vi "Auto Build Script.vi"(8 "error in (no error)":errorcluster, 11 "PostBuildSupport":refnum<class "PostBuildSupport.lvclass">) -> (0 "error out":errorcluster)   [LabVIEW 2019, in "PostBuildSupport.lvclass"]
uses:
  PostBuildSupport.lvclass
  <userlib>/LevyLab/Progress Bar/ProgressBar/ProgressBar.lvclass
panel:
  in  "OK":bool
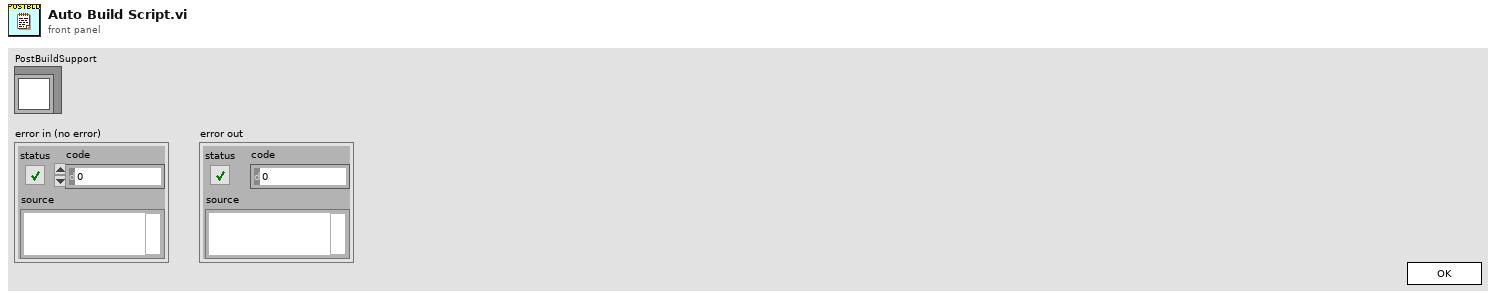
[diagram p1: front panel]
types:
  T1 = enum32{"Invalid", "Standard", "Closed", "Hidden", "Minimized", "Maximized"}
  T2 = enum32{"invalid app kind", "Development System", "Run Time System", "Student Edition", "Embedded LabVIEW", "Evaluation", "Custom"}
  T3 = cluster{"Core":cluster{"Current VI Reference":refnum<vi>, "Close Panel on Exit?":bool}, "PostBuildSupport":refnum<class "PostBuildSupport.lvclass">, "ProgressBar out":refnum<class "ProgressBar.lvclass">, "Progress Message":string, "Progress Bar":i32}
  T4 = cluster{"Current VI Reference":refnum<vi>, "Close Panel on Exit?":bool}
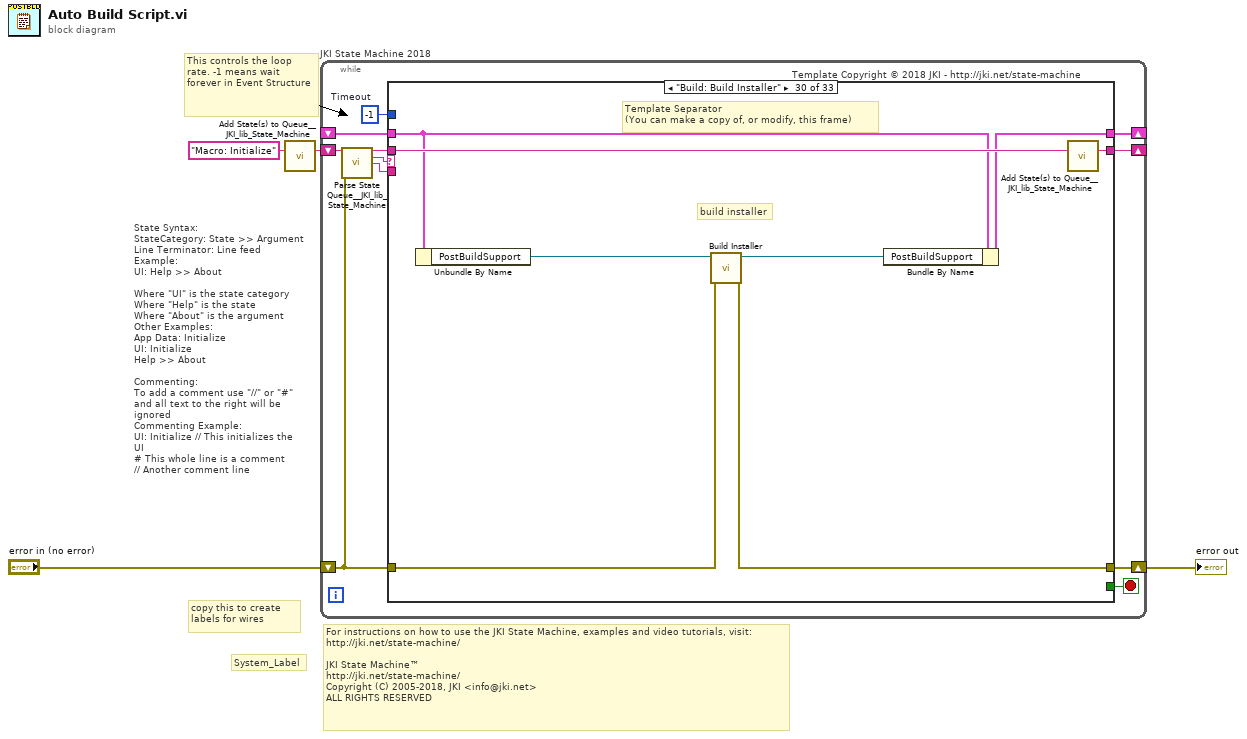
[diagram p0: block diagram]
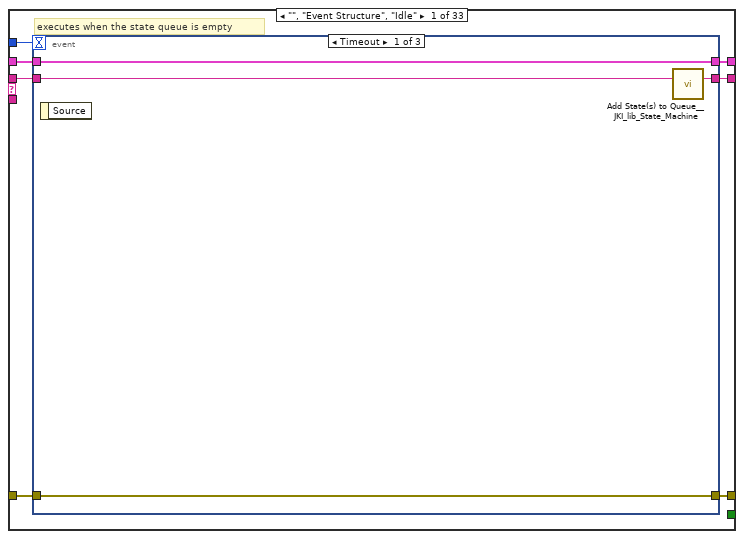
[diagram p2: hidden frame]
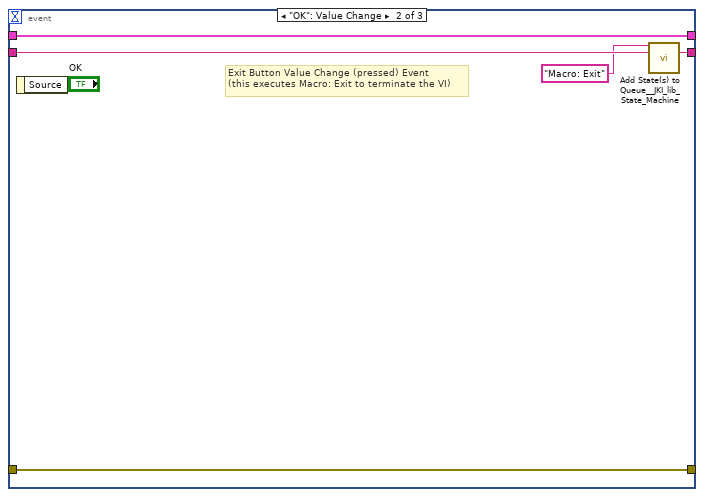
[diagram p3: hidden frame]
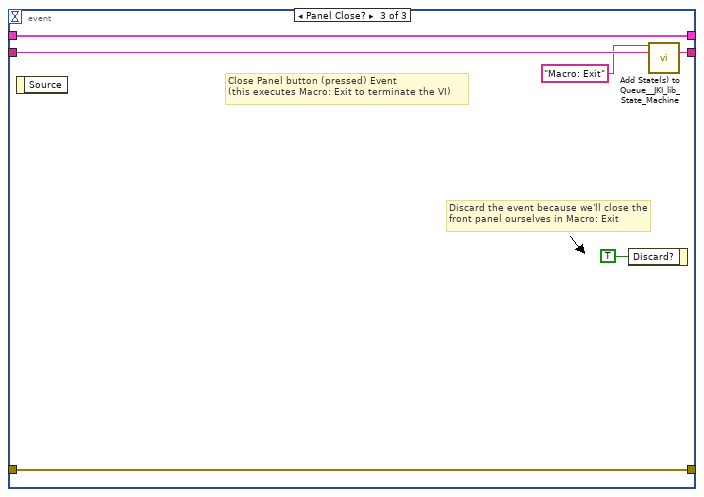
[diagram p4: hidden frame]
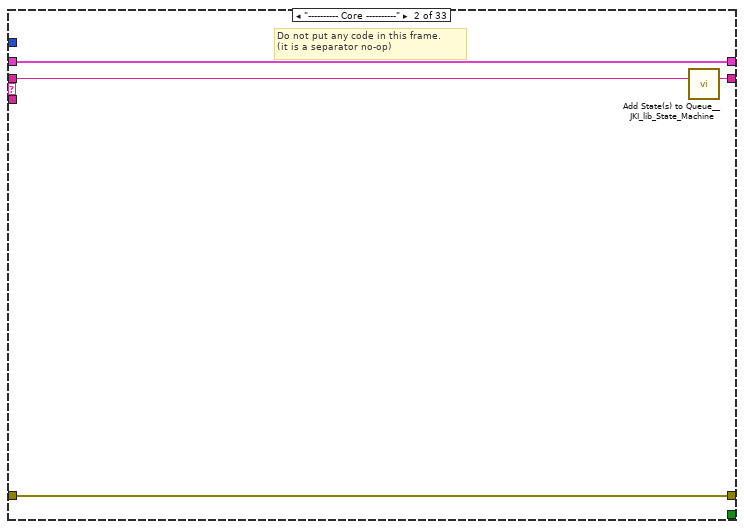
[diagram p5: hidden frame]
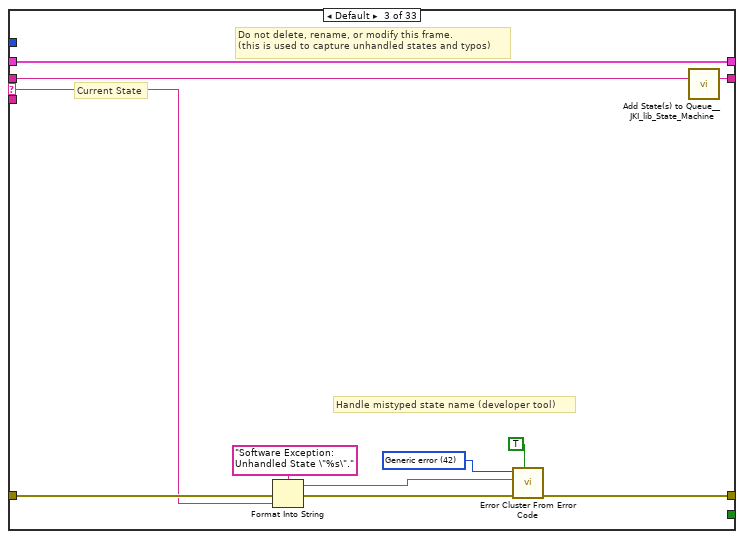
[diagram p6: hidden frame]
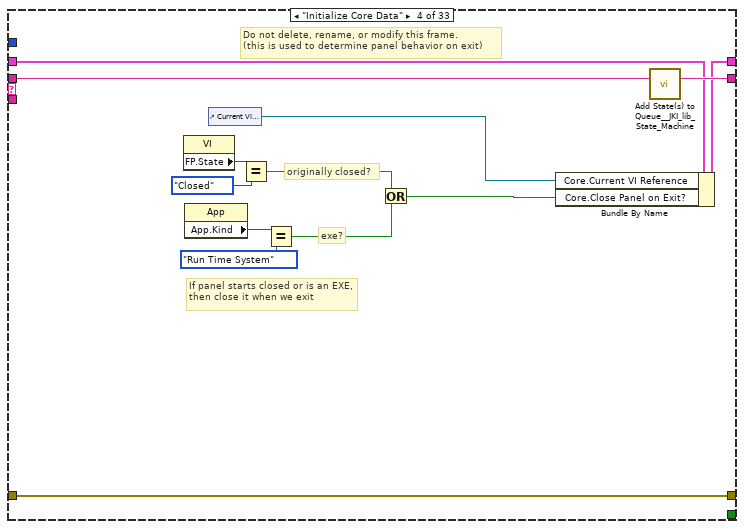
[diagram p7: hidden frame]
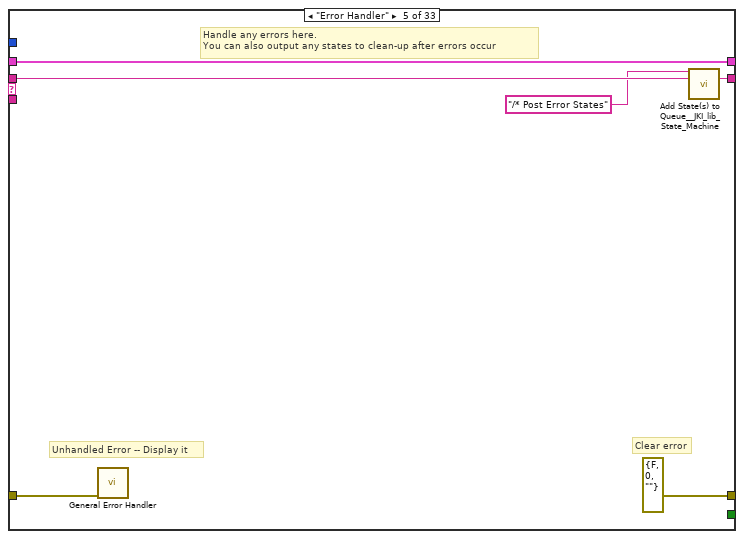
[diagram p8: hidden frame]
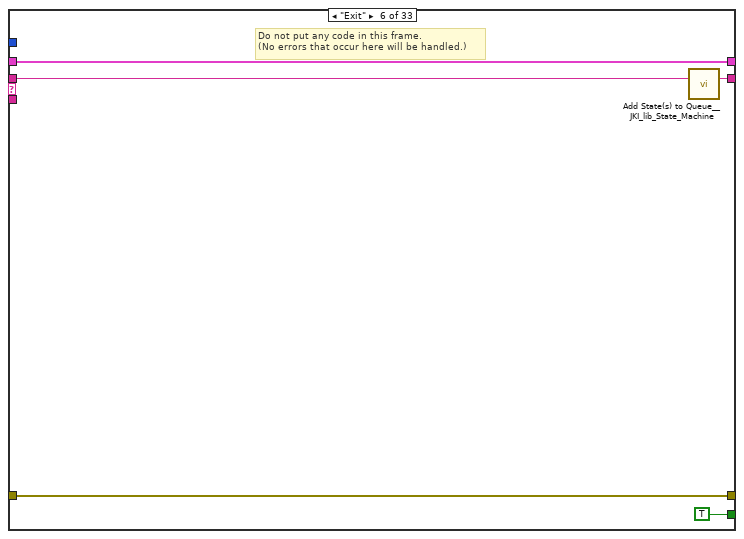
[diagram p9: hidden frame]
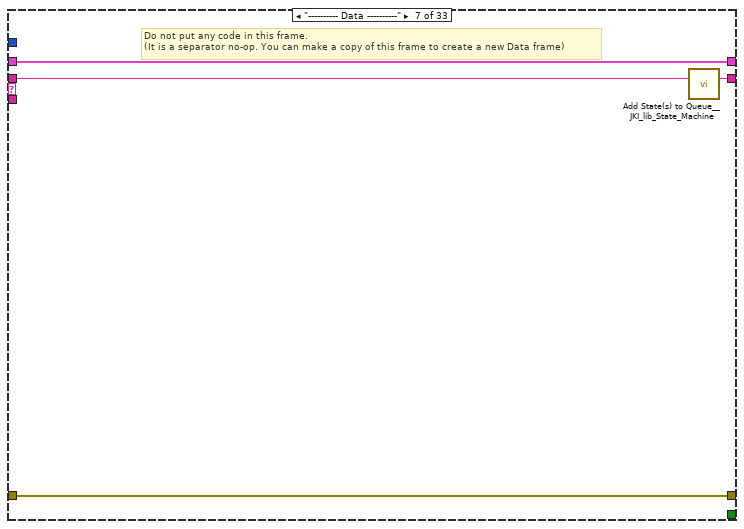
[diagram p10: hidden frame]
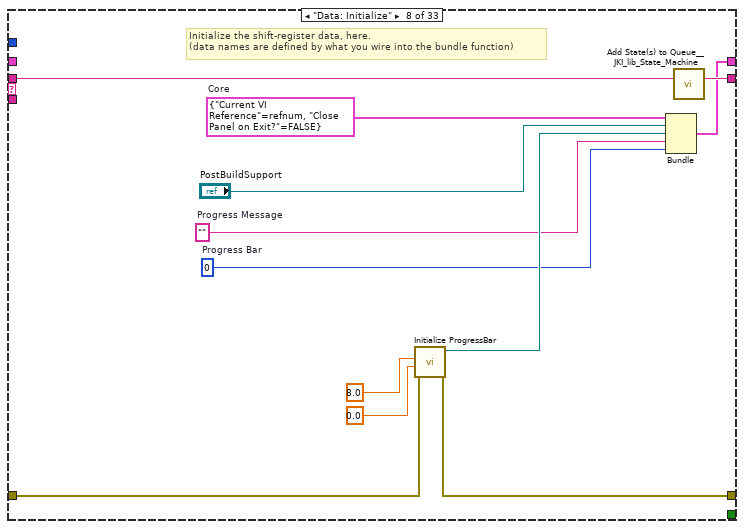
[diagram p11: hidden frame]
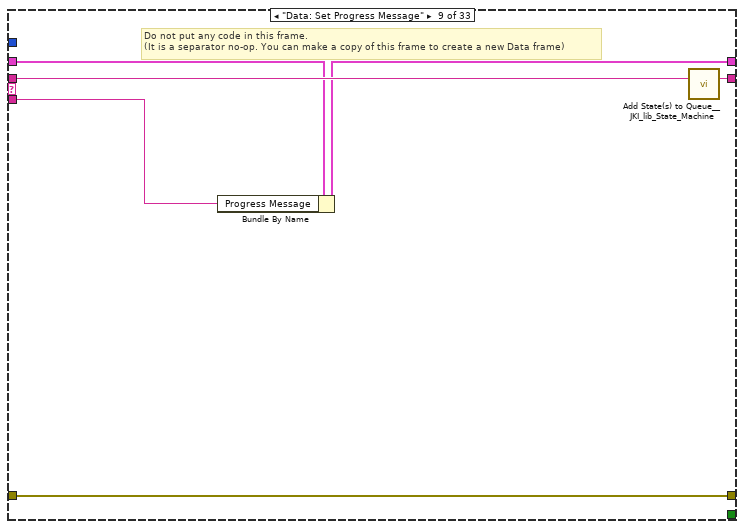
[diagram p12: hidden frame]
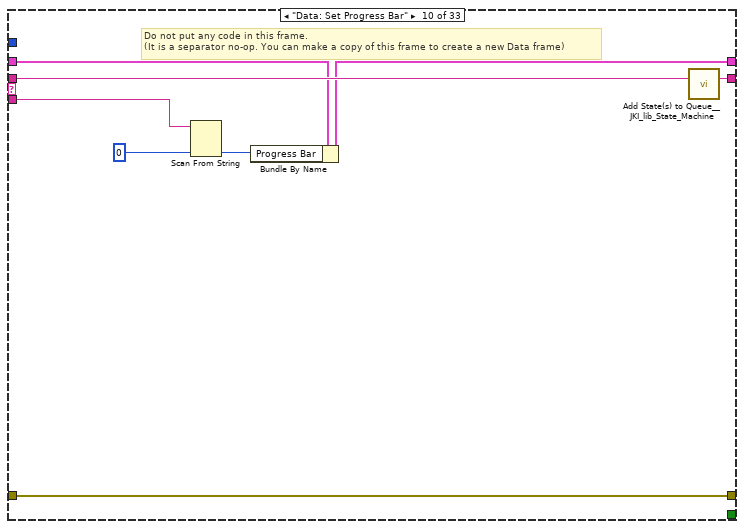
[diagram p13: hidden frame]
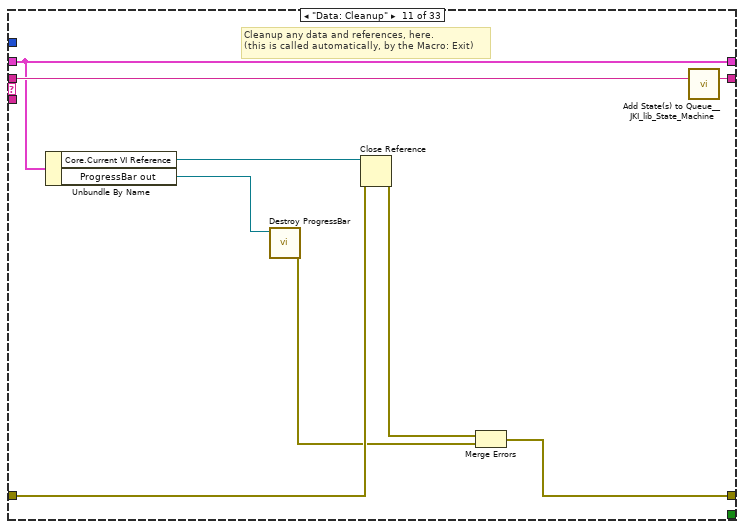
[diagram p14: hidden frame]
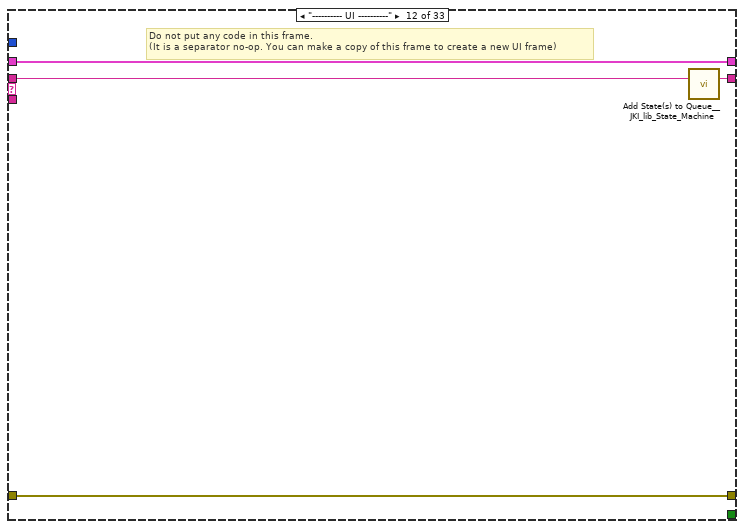
[diagram p15: hidden frame]
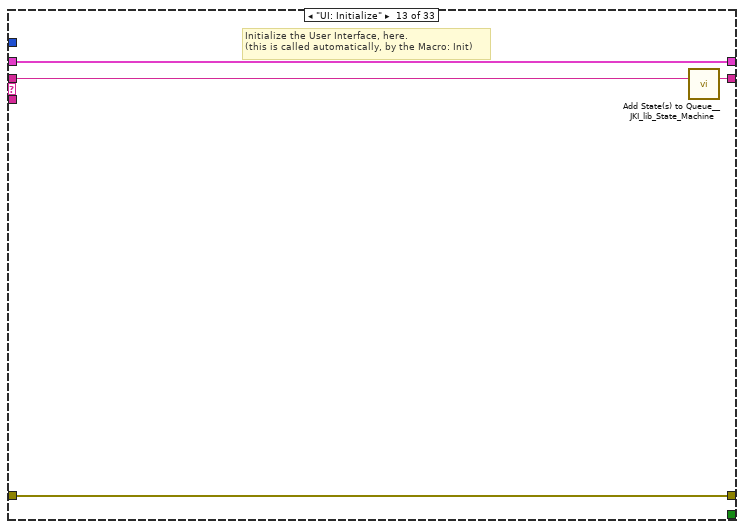
[diagram p16: hidden frame]
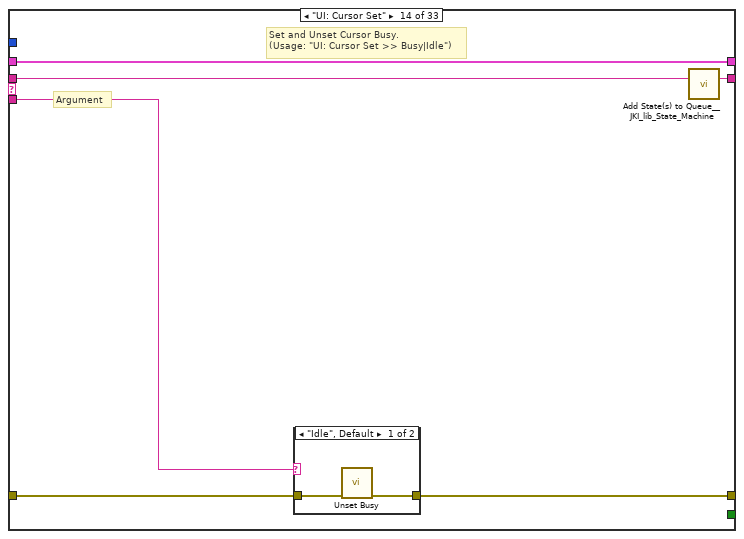
[diagram p17: hidden frame]
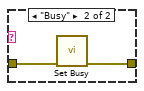
[diagram p18: hidden frame]
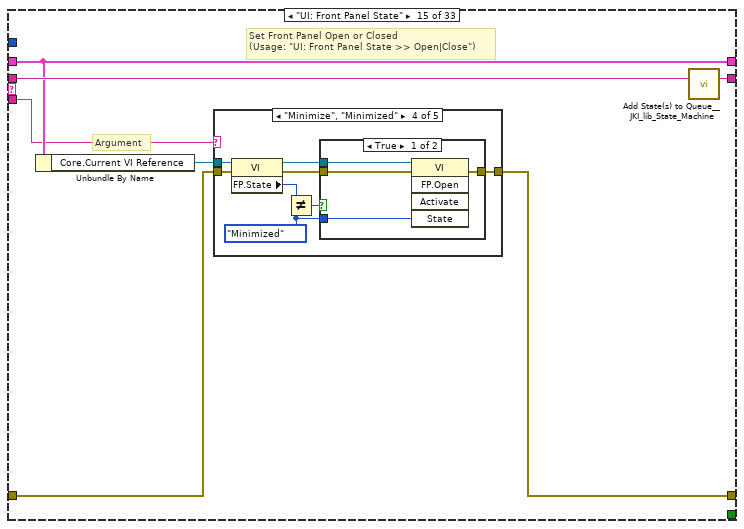
[diagram p19: hidden frame]
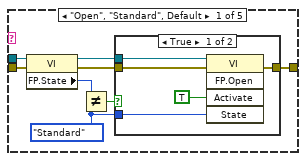
[diagram p20: hidden frame]
diagram:
  # "For instructions on how to use the JKI State Machine, examples and video tutorials, visit:\nhttp://jki.net/state-machine/\n\nJKI State Machine™\nhttp://jki.net/state-machine/\nCopyright (C) 2005-2018, JKI <info@jki.net>\nALL RIGHTS RESERVED"
  # "State Syntax:\nStateCategory: State >> Argument\nLine Terminator: Line feed\nExample:\nUI: Help >> About\n\nWhere \"UI\" is the state category\nWhere \"Help\" is the state\nWhere \"About\" is the argument\nOther Examples:\nApp Data: Initialize\nUI: Initialize\nHelp >> About\n\nCommenting:\nTo add a comment use \"//\" or \"#\" and all text to the right will be ignored\nCommenting Example:\nUI: Initialize // This initializes the UI\n# This whole line is a comment\n// Another comment line"
  # "copy this to create labels for wires"
  # "This controls the loop rate. -1 means wait forever in Event Structure"
  # "System_Label"
  n1 = call <vilib>:"Add State(s) to Queue__JKI_lib_State_Machine.vi"("State(s) in (\"\")"="Macro: Initialize") -> ("States Out"=w4:string)  [unwired: 14 in]
  n2 = while "JKI State Machine 2018" {
    shift-right: [w8] -> _
    shift-left: _ -> [w7]
    shift-right: [w11] -> w1
    shift-left: "error in (no error)" -> [w5]
    shift-right: [w10] -> _
    shift-left: w4 -> [w12]
    stop <- w9 stop-if-true
    w6 = -1  # Timeout
    # "Template Copyright © 2018 JKI - http://jki.net/state-machine"
    n3 = call <vilib>:"Parse State Queue__JKI_lib_State_Machine.vi"("State Queue"=w12, "Error In (no error)"=w5) -> ("Remaining States"=w14:string, "Current State"=w15:string, "Arguments"=w13:string)  [unwired: 11 in]
    n4 = case shown="\"Build: Build Installer\"" w15 {
      selector: w15 -> [_ _ w42 _ _ _ _ _ _ _ _ _ _ _ _ _ _ _ _ _ _ _ _ _ _ _ _ _ _ _ _ _ _]
      tunnel: w14 -> [w22 w41 w46 w65 w71 w76 w80 w92 w98 w106 w115 w119 w123 w129 w140 w209 w214 w219 w224 w234 w238 w248 w254 w260 w268 w276 w284 w292 w300 w308 w316 w324 w332]
      tunnel: w13 -> [_ _ _ _ _ _ _ _ w95 w100 _ _ _ w124 w134 _ _ _ _ _ _ _ _ _ _ _ _ _ _ _ _ _ _]
      tunnel: w7 -> [w20 w38 w44 w58 w68 w74 w77 _ w93 w102 w112 w116 w121 w127 w136 w206 w211 w216 w221 w231 w235 w244 w250 w256 w265 w273 w281 w289 w297 w305 w313 w321 w329]
      tunnel: [w19 w39 w48 w62 errorcluster {"status"=FALSE, "code"=0, "source"=""} ("error out") w73 w78 w86 w96 w104 w108 w117 w120 w125 w137 w207 w212 w217 w222 w232 w236 w240 w252 w258 w264 w272 w278 w287 w296 w301 w311 w320 w327] -> w11
      tunnel: w5 -> [w18 w39 w47 w62 w67 w73 w78 w85 w96 w104 w110 w117 w120 w126 w138 w207 w212 w217 w222 w232 w236 w239 w252 w258 w261 w269 w277 w286 w294 w302 w310 w317 w326]
      tunnel: [w21 w40 w45 w64 w70 w75 w79 w91 w97 w105 w114 w118 w122 w128 w139 w208 w213 w218 w223 w233 w237 w247 w253 w259 w267 w275 w283 w291 w299 w307 w315 w323 w331] -> w10
      tunnel: [_ _ _ _ _ TRUE _ _ _ _ _ _ _ _ _ _ _ _ _ _ _ _ _ _ _ _ _ _ _ _ _ _ _] -> w9
      tunnel: [w17 w38 w44 w63 w68 w74 w77 w81 w94 w103 w112 w116 w121 w127 w136 w206 w211 w216 w221 w231 w235 w244 w251 w257 w266 w274 w282 w290 w298 w306 w314 w322 w330] -> w8
      tunnel: w6 -> [w16 _ _ _ _ _ _ _ _ _ _ _ _ _ _ _ _ _ _ _ _ _ _ _ _ _ _ _ _ _ _ _ _]
      frame "", "Event Structure", "Idle" {
        # "executes when the state queue is empty"
        n5 = event shown="[0] Timeout" {
          selector: _ -> [_ _ _]
          dyn-events: _ -> [_ _ _]
          timeout: w16 -> [_ _ _]
          tunnel: w22 -> [w26 w31 w37]
          tunnel: [w25 w30 w36] -> w21
          tunnel: w20 -> [w23 w28 w34]
          tunnel: [w24 w29 w35] -> w19
          tunnel: w18 -> [w24 w29 w35]
          tunnel: [w23 w28 w34] -> w17
          event Timeout {
            n6 = event-data() -> ()  [unwired: 1 in, 1 out]
            n7 = call <vilib>:"Add State(s) to Queue__JKI_lib_State_Machine.vi"("State(s) in (\"\")"=w26) -> ("States Out"=w25:string)  [unwired: 14 in]
          }
          event "OK": Value Change {
            # "Exit Button Value Change (pressed) Event\n(this executes Macro: Exit to terminate the VI)"
            n8 = event-data() -> ()  [unwired: 1 in, 1 out]
            n9 = call <vilib>:"Add State(s) to Queue__JKI_lib_State_Machine.vi"("State(s) in Front (\"\")"="Macro: Exit", "State(s) in (\"\")"=w31) -> ("States Out"=w30:string)  [unwired: 13 in]
          }
          event Panel Close? {
            # "Discard the event because we'll close the front panel ourselves in Macro: Exit"
            # "Close Panel button (pressed) Event\n(this executes Macro: Exit to terminate the VI)"
            n10 = event-data() -> ()  [unwired: 1 in, 1 out]
            n11 = event-data("Discard?"=TRUE) -> ()  [unwired: 1 in, 1 out]
            n12 = call <vilib>:"Add State(s) to Queue__JKI_lib_State_Machine.vi"("State(s) in Front (\"\")"="Macro: Exit", "State(s) in (\"\")"=w37) -> ("States Out"=w36:string)  [unwired: 13 in]
          }
        }
      }
      frame "---------- Core ----------" {
        # "Do not put any code in this frame.\n(it is a separator no-op)"
        n13 = call <vilib>:"Add State(s) to Queue__JKI_lib_State_Machine.vi"("State(s) in (\"\")"=w41) -> ("States Out"=w40:string)  [unwired: 14 in]
      }
      frame Default {
        w51 = 42 items=["No error", "Argument error", "Memory is full", "Out of zone", "End of file", "File already open", "Generic file I/O error", "File not found", "File permission error", "Disk is full", "Duplicate path", "Too many files open", "System feature not enabled", "Resource file not found", "Cannot add resource", "Resource not found", "Image not found", "Image memory error", "Pen does not exist", "Config type invalid", "Config token not found", "Config parse error", "Config memory error", "Bad external code format", "Bad external code offset", "External code not present", "Null window", "Destroy window error", "Null menu", "Print aborted", "Bad print record", "Print driver error", "Windows error during printing", "Memory error during printing", "Print dialog error", "Generic print error", "Invalid device refnum", "Device not found", "Device parameter error", "Device unit error", "Cannot open device", "Device call aborted", "Generic error", "Cancelled by user", "Object ID too low", "Object ID too high", "Object not in heap", "Unknown heap", "Unknown object (invalid DefProc)", "Unknown object (DefProc not in table)", "Message out of range", "Invalid (null) method", "Unknown message", "Manager call not supported", "Bad address", "Network operation in progress", "Network operation timed out", "Connection is busy", "Network attribute not supported", "Network error", "Address in use", "System out of memory", "Connection aborted", "Connection refused", "Not connected", "Already connected", "Connection closed", "Initialization error (interapplication manager)", "Bad occurrence", "Wait on unbound occurrence handler", "Occurrence queue overflow", "Datalog type conflict", "Unused", "Unrecognized type (interapplication manager)", "Memory corrupt", "Failed to make temporary DLL", "Old CIN version", "Drag socket not found", "Failed to load drop-object", "Failed to register OLE object", "Failed to release OLE object", "Format specifier type mismatch", "Unknown format specifier", "Too few format specifiers", "Too many format specifiers", "Scan failed", "Newer CIN version", "Error converting to variant", "Runtime menu error", "Password tampered", "Variant attribute not found", "Incompatible variant data type", "Event data is not available", "Event Store is not present", "Occurrence is not found", "Event Queue is not created", "Event info is not available", "Refnum passed is NULL", "Error retrieving Class GUID", "Error retrieving CoClass GUID", "Error retrieving TypeLib GUID.", "Bad built application magic bytes.", "Specific driver is different from the specific driver associated with the Logical Name.", "There is no session opened to the class driver.", "Max Error", "MAX - Error with config objects", "MAX - Error loading configuration", "MAX - Group not supported"]
        # "Current State"
        # "Do not delete, rename, or modify this frame.\n(this is used to capture unhandled states and typos)"
        # "Handle mistyped state name (developer tool)"
        n14 = Format Into String(format string="Software Exception: Unhandled State \"%s\"." ("message"), error in=w47, w42) -> (resulting string=w50:string, error out=w49:errorcluster)  [unwired: 1 in]
        n15 = call <vilib>:"Error Cluster From Error Code.vi"("show call chain? (False)"=TRUE, "error in (no error)"=w49, "error message (\"\")"=w50, "error code (0)"=w51) -> ("error out"=w48:errorcluster)  [unwired: 5 in]
        n16 = call <vilib>:"Add State(s) to Queue__JKI_lib_State_Machine.vi"("State(s) in (\"\")"=w46) -> ("States Out"=w45:string)  [unwired: 14 in]
      }
      frame "Initialize Core Data" {
        # "Do not delete, rename, or modify this frame.\n(this is used to determine panel behavior on exit)"
        # "originally closed?"
        # "exe?"
        # "If panel starts closed or is an EXE, then close it when we exit"
        n17 = property class="VI"() -> ("FP.State"=w55:T1)  [unwired: 2 in, 2 out]
        n18 = property class="App"() -> ("App.Kind"=w61:T2)  [unwired: 2 in, 2 out]
        n19 = control-ref of="Current VI Reference"() -> (w56:refnum<vi>)
        n20 = Equal?(x=w55, y=T1."Closed" ("Front Panel Window:State")) -> (x = y?=w53:bool)
        n21 = Equal?(x=w61, y=T2."Run Time System" ("Application:Kind")) -> (x = y?=w59:bool)
        n22 = Or(x=w53, y=w59) -> (x .or. y?=w57:bool)
        n23 = Bundle By Name(cluster=w58, "Core.Current VI Reference"=w56, "Core.Close Panel on Exit?"=w57) -> (w63:T3)
        n24 = call <vilib>:"Add State(s) to Queue__JKI_lib_State_Machine.vi"("State(s) in (\"\")"=w65) -> ("States Out"=w64:string)  [unwired: 14 in]
      }
      frame "Error Handler" {
        # "Unhandled Error -- Display it"
        # "Handle any errors here.\nYou can also output any states to clean-up after errors occur"
        # "Clear error"
        n25 = call <vilib>:"General Error Handler.vi"("error in (no error)"=w67) -> ()  [unwired: 10 in, 5 out]
        n26 = call <vilib>:"Add State(s) to Queue__JKI_lib_State_Machine.vi"("State(s) in Front (\"\")"="/* Post Error States", "State(s) in (\"\")"=w71) -> ("States Out"=w70:string)  [unwired: 13 in]
      }
      frame "Exit" {
        # "Do not put any code in this frame.\n(No errors that occur here will be handled.)"
        n27 = call <vilib>:"Add State(s) to Queue__JKI_lib_State_Machine.vi"("State(s) in (\"\")"=w76) -> ("States Out"=w75:string)  [unwired: 14 in]
      }
      frame "---------- Data ----------" {
        # "Do not put any code in this frame.\n(It is a separator no-op. You can make a copy of this frame to create a new Data frame)"
        n28 = call <vilib>:"Add State(s) to Queue__JKI_lib_State_Machine.vi"("State(s) in (\"\")"=w80) -> ("States Out"=w79:string)  [unwired: 14 in]
      }
      frame "Data: Initialize" {
        w90 = T4 {"Current VI Reference"=refnum, "Close Panel on Exit?"=FALSE}  # Core
        w82 = 0  # Progress Bar
        w83 = ""  # Progress Message
        # "Initialize the shift-register data, here.\n(data names are defined by what you wire into the bundle function)"
        n29 = call <userlib>:"Initialize ProgressBar.vi"("error in (no error)"=w85, "Scale Min"=0.0 ("Min (0)"), "Scale Max"=8.0 ("Max (1)")) -> ("error out"=w86:errorcluster, "ProgressBar out"=w84:refnum<class "ProgressBar.lvclass">)  [unwired: 7 in]
        n30 = Bundle("Core"=w90, "PostBuildSupport"="PostBuildSupport", "ProgressBar out"=w84, "Progress Message"=w83, "Progress Bar"=w82) -> (w81:T3)  [unwired: 1 in]
        n31 = call <vilib>:"Add State(s) to Queue__JKI_lib_State_Machine.vi"("State(s) in (\"\")"=w92) -> ("States Out"=w91:string)  [unwired: 14 in]
      }
      frame "Data: Set Progress Message" {
        # "Do not put any code in this frame.\n(It is a separator no-op. You can make a copy of this frame to create a new Data frame)"
        n32 = Bundle By Name(cluster=w93, "Progress Message"=w95) -> (w94:T3)
        n33 = call <vilib>:"Add State(s) to Queue__JKI_lib_State_Machine.vi"("State(s) in (\"\")"=w98) -> ("States Out"=w97:string)  [unwired: 14 in]
      }
      frame "Data: Set Progress Bar" {
        # "Do not put any code in this frame.\n(It is a separator no-op. You can make a copy of this frame to create a new Data frame)"
        n34 = Scan From String(input string=w100, default 1=0 ("Progress Bar")) -> (output 1=w99:i32)  [unwired: 3 in, 3 out]
        n35 = Bundle By Name(cluster=w102, "Progress Bar"=w99) -> (w103:T3)
        n36 = call <vilib>:"Add State(s) to Queue__JKI_lib_State_Machine.vi"("State(s) in (\"\")"=w106) -> ("States Out"=w105:string)  [unwired: 14 in]
      }
      frame "Data: Cleanup" {
        # "Cleanup any data and references, here.\n(this is called automatically, by the Macro: Exit)"
        n37 = Unbundle By Name(w112) -> ("Core.Current VI Reference"=w113:refnum<vi>, "ProgressBar out"=w111:refnum<class "ProgressBar.lvclass">)
        n38 = call <userlib>:"Destroy ProgressBar.vi"("ProgressBar in"=w111) -> ("error out"=w109:errorcluster)  [unwired: 9 in, 1 out]
        n39 = Close Reference(reference=w113, error in (no error)=w110) -> (error out=w107:errorcluster)
        n40 = Merge Errors(w107, w109) -> (w108:errorcluster)
        n41 = call <vilib>:"Add State(s) to Queue__JKI_lib_State_Machine.vi"("State(s) in (\"\")"=w115) -> ("States Out"=w114:string)  [unwired: 14 in]
      }
      frame "---------- UI ----------" {
        # "Do not put any code in this frame.\n(It is a separator no-op. You can make a copy of this frame to create a new UI frame)"
        n42 = call <vilib>:"Add State(s) to Queue__JKI_lib_State_Machine.vi"("State(s) in (\"\")"=w119) -> ("States Out"=w118:string)  [unwired: 14 in]
      }
      frame "UI: Initialize" {
        # "Initialize the User Interface, here.\n(this is called automatically, by the Macro: Init)"
        n43 = call <vilib>:"Add State(s) to Queue__JKI_lib_State_Machine.vi"("State(s) in (\"\")"=w123) -> ("States Out"=w122:string)  [unwired: 14 in]
      }
      frame "UI: Cursor Set" {
        # "Argument"
        # "Set and Unset Cursor Busy.\n(Usage: \"UI: Cursor Set >> Busy|Idle\")"
        n44 = case shown="\"Idle\", Default" w124 {
          tunnel: w126 -> [w131 w133]
          tunnel: [w130 w132] -> w125
          frame "Idle", Default {
            n45 = call <vilib>:"Unset Busy.vi"("error in (no error)"=w131) -> ("error out"=w130:errorcluster)  [unwired: 10 in]
          }
          frame "Busy" {
            n46 = call <vilib>:"Set Busy.vi"("error in (no error)"=w133) -> ("error out"=w132:errorcluster)  [unwired: 9 in, 1 out]
          }
        }
        n47 = call <vilib>:"Add State(s) to Queue__JKI_lib_State_Machine.vi"("State(s) in (\"\")"=w129) -> ("States Out"=w128:string)  [unwired: 14 in]
      }
      frame "UI: Front Panel State" {
        # "Argument"
        # "Set Front Panel Open or Closed\n(Usage: \"UI: Front Panel State >> Open|Close\")"
        n48 = Unbundle By Name(w136) -> ("Core.Current VI Reference"=w135:refnum<vi>)
        n49 = case shown="\"Minimize\", \"Minimized\"" w134 {
          tunnel: w138 -> [w146 w161 w172 w185 w198]
          tunnel: [w148 w162 w174 w187 w200] -> w137
          tunnel: w135 -> [w147 w159 w173 w186 w199]
          frame "Open", "Standard", Default {
            w141 = T1."Standard" ("State")
            n50 = property class="VI"(reference=w147, error in=w146) -> (reference out=w144:refnum<vi>, error out=w145:errorcluster, "FP.State"=w143:T1)
            n51 = Not Equal?(x=w143, y=w141) -> (x != y?=w142:bool)
            n52 = case shown="True" w142 {
              tunnel: [w152 w154] -> w148
              tunnel: w145 -> [w151 w154]
              tunnel: w144 -> [w150 _]
              tunnel: w141 -> [w149 _]
              frame True {
                n53 = invoke class="VI" method="FP.Open"(reference=w150, error in=w151, "Activate"=TRUE, "State"=w149) -> (error out=w152:errorcluster)  [unwired: 1 in, 4 out]
              }
              frame False {
              }
            }
          }
          frame "Close", "Closed" {
            n54 = property class="VI"(reference=w159, error in=w161) -> (reference out=w158:refnum<vi>, error out=w160:errorcluster, "FP.State"=w156:T1)
            n55 = Not Equal?(x=w156, y=T1."Closed" ("Front Panel Window:State")) -> (x != y?=w155:bool)
            n56 = case shown="True" w155 {
              tunnel: [w163 w166] -> w162
              tunnel: w160 -> [w163 w165]
              tunnel: w158 -> [_ w164]
              frame False {
              }
              frame True {
                n57 = invoke class="VI" method="FP.Close"(reference=w164, error in=w165) -> (error out=w166:errorcluster)  [unwired: 1 in, 2 out]
              }
            }
          }
          frame "Hidden", "Hide" {
            w167 = T1."Hidden" ("State")
            n58 = property class="VI"(reference=w173, error in=w172) -> (reference out=w170:refnum<vi>, error out=w171:errorcluster, "FP.State"=w169:T1)
            n59 = Not Equal?(x=w169, y=w167) -> (x != y?=w168:bool)
            n60 = case shown="True" w168 {
              tunnel: [w178 w179] -> w174
              tunnel: w171 -> [w177 w179]
              tunnel: w170 -> [w176 _]
              tunnel: w167 -> [w175 _]
              frame True {
                n61 = invoke class="VI" method="FP.Open"(reference=w176, error in=w177, "State"=w175) -> (error out=w178:errorcluster)  [unwired: 2 in, 4 out]
              }
              frame False {
              }
            }
          }
          frame "Minimize", "Minimized" {
            w180 = T1."Minimized" ("State")
            n62 = property class="VI"(reference=w186, error in=w185) -> (reference out=w183:refnum<vi>, error out=w184:errorcluster, "FP.State"=w182:T1)
            n63 = Not Equal?(x=w182, y=w180) -> (x != y?=w181:bool)
            n64 = case shown="True" w181 {
              tunnel: [w191 w192] -> w187
              tunnel: w184 -> [w190 w192]
              tunnel: w183 -> [w189 _]
              tunnel: w180 -> [w188 _]
              frame True {
                n65 = invoke class="VI" method="FP.Open"(reference=w189, error in=w190, "State"=w188) -> (error out=w191:errorcluster)  [unwired: 2 in, 4 out]
              }
              frame False {
              }
            }
          }
          frame "Maximize", "Maximized" {
            w193 = T1."Maximized" ("State")
            n66 = property class="VI"(reference=w199, error in=w198) -> (reference out=w196:refnum<vi>, error out=w197:errorcluster, "FP.State"=w195:T1)
            n67 = Not Equal?(x=w195, y=w193) -> (x != y?=w194:bool)
            n68 = case shown="True" w194 {
              tunnel: [w204 w205] -> w200
              tunnel: w197 -> [w203 w205]
              tunnel: w196 -> [w202 _]
              tunnel: w193 -> [w201 _]
              frame True {
                n69 = invoke class="VI" method="FP.Open"(reference=w202, error in=w203, "State"=w201) -> (error out=w204:errorcluster)  [unwired: 2 in, 4 out]
              }
              frame False {
              }
            }
          }
        }
        n70 = call <vilib>:"Add State(s) to Queue__JKI_lib_State_Machine.vi"("State(s) in (\"\")"=w140) -> ("States Out"=w139:string)  [unwired: 14 in]
      }
      frame "---------- Macro ----------" {
        # "Do not put any code in this frame.\n(It is a separator no-op. You can make a copy of this frame to create a new Macro frame)"
        n71 = call <vilib>:"Add State(s) to Queue__JKI_lib_State_Machine.vi"("State(s) in (\"\")"=w209) -> ("States Out"=w208:string)  [unwired: 14 in]
      }
      frame "Macro: Initialize" {
        # "Initialization Macro\n(This is called once, when the VI starts)"
        n72 = call <vilib>:"Add State(s) to Queue__JKI_lib_State_Machine.vi"("State(s) in Front (\"\")"="Data: Initialize\nInitialize Core Data\nUI: Initialize\nUI: Front Panel State >> Close\nMacro: Prepare Build\nMacro: Build\nMacro: Exit", "State(s) in (\"\")"=w214) -> ("States Out"=w213:string)  [unwired: 13 in]
      }
      frame "Macro: Prepare Build" {
        # "Do not put any code in this frame.\n(It is a separator no-op. You can make a copy of this frame to create a new Macro frame)"
        n73 = call <vilib>:"Add State(s) to Queue__JKI_lib_State_Machine.vi"("State(s) in Front (\"\")"="Data: Set Progress Message >> Setting up Folder Structure\nData: Set Progress Bar >> 0\nBuild: Setup Folder Structure\n\nData: Set Progress Message >> Copy Latest VIP File\nData: Set Progress Bar >> 1\nBuild: Copy Latest VIP File\n\nData: Set Progress Message >> Copy 7zSD.sfx\nData: Set Progress Bar >> 2\nBuild: Copy 7zSD\n\nData: Set Progress Message >> Loading LV Project\nData: Set Progress Bar >> 3\nBuild: Load LV Project\n\nData: Set Progress Message >> Update Build Version\nData: Set Progress Bar >> 4\nBuild: Update Build Version" ("State(s) in Front (\"\")"), "State(s) in (\"\")"=w219) -> ("States Out"=w218:string)  [unwired: 13 in]
      }
      frame "Macro: Build" {
        # "Do not put any code in this frame.\n(It is a separator no-op. You can make a copy of this frame to create a new Macro frame)"
        n74 = call <vilib>:"Add State(s) to Queue__JKI_lib_State_Machine.vi"("State(s) in Front (\"\")"="Data: Set Progress Message >> Building Application\nData: Set Progress Bar >> 5\nBuild: Build Application\n\nData: Set Progress Message >> Building Installer\nData: Set Progress Bar >> 6\nBuild: Build Installer\n\nData: Set Progress Message >> Writing 7z Config.txt\nData: Set Progress Bar >> 7\nBuild: Write 7z Config\n\nData: Set Progress Message >> Writing 7z.bat\nData: Set Progress Bar >> 8\nBuild: Write 7z\n\nData: Set Progress Message >> Writing 7z.bat\nData: Set Progress Bar >> 9\nBuild: Execute 7z" ("State(s) in Front (\"\")"), "State(s) in (\"\")"=w224) -> ("States Out"=w223:string)  [unwired: 13 in]
      }
      frame "Macro: Exit" {
        # "Exit Macro\n(This is called once, when the VI exits)"
        n75 = Unbundle By Name(w231) -> ("Core.Close Panel on Exit?"=w230:bool)
        n76 = Select(t="UI: Front Panel State >> Close", s=w230, f="") -> (s? t:f=w227:string)
        n77 = call <vilib>:"Add State(s) to Queue__JKI_lib_State_Machine.vi"("State(s) in (\"\")"=w227, "State(s) at Back (\"\")"="Data: Cleanup\nExit") -> ("States Out"=w225:string)  [unwired: 13 in]
        n78 = call <vilib>:"Add State(s) to Queue__JKI_lib_State_Machine.vi"("State(s) in Front (\"\")"=w225, "State(s) in (\"\")"=w234) -> ("States Out"=w233:string)  [unwired: 13 in]
      }
      frame "---------- Progress ----------" {
        # "Template Separator\n(You can make a copy of, or modify, this frame)"
        n79 = call <vilib>:"Add State(s) to Queue__JKI_lib_State_Machine.vi"("State(s) in (\"\")"=w238) -> ("States Out"=w237:string)  [unwired: 14 in]
      }
      frame "Progress: Update" {
        # "Your code here.\n(You can make a copy of, or modify, this frame)"
        n80 = Unbundle By Name(w244) -> ("ProgressBar out"=w243:refnum<class "ProgressBar.lvclass">, "Progress Message"=w242:string, "Progress Bar"=w241:i32)
        n81 = call <userlib>:"Send Progress and Message.vi"("error in (no error)"=w239, "Progress"=w241, "Message"=w242, "ProgressBar in"=w243) -> ("error out"=w245:errorcluster)  [unwired: 6 in, 1 out]
        n82 = call <userlib>:"Wait (ms)__ogtk.vi"("error in (no error)"=w245, "milliseconds to wait"=u32 200) -> ("error out"=w240:errorcluster)  [unwired: 8 in, 1 out]
        n83 = call <vilib>:"Add State(s) to Queue__JKI_lib_State_Machine.vi"("State(s) in (\"\")"=w248) -> ("States Out"=w247:string)  [unwired: 14 in]
      }
      frame "---------- Build ----------" {
        # "Template Separator\n(You can make a copy of, or modify, this frame)"
        n84 = Unbundle By Name(w250) -> ("PostBuildSupport"=w249:refnum<class "PostBuildSupport.lvclass">)
        n85 = Bundle By Name(cluster=w250, "PostBuildSupport"=w249) -> (w251:T3)
        n86 = call <vilib>:"Add State(s) to Queue__JKI_lib_State_Machine.vi"("State(s) in (\"\")"=w254) -> ("States Out"=w253:string)  [unwired: 14 in]
      }
      frame "Build: Setup Folder Structure" {
        # "setup up folder structure \n(if doesn't exist already)"
        # "Template Separator\n(You can make a copy of, or modify, this frame)"
        n87 = Unbundle By Name(w256) -> ("PostBuildSupport"=w255:refnum<class "PostBuildSupport.lvclass">)
        n88 = call "Create Folders.vi"() -> ()  [unwired: 10 in, 2 out]
        n89 = Bundle By Name(cluster=w256, "PostBuildSupport"=w255) -> (w257:T3)
        n90 = call <vilib>:"Add State(s) to Queue__JKI_lib_State_Machine.vi"("State(s) in (\"\")"=w260) -> ("States Out"=w259:string)  [unwired: 14 in]
      }
      frame "Build: Copy Latest VIP File" {
        # "copy latest vip file"
        n91 = Unbundle By Name(w265) -> ("PostBuildSupport"=w263:refnum<class "PostBuildSupport.lvclass">)
        n92 = call "Copy Package.vi"("error in (no error)"=w261, "PostBuildSupport in"=w263) -> ("error out"=w264:errorcluster, "PostBuildSupport out"=w262:refnum<class "PostBuildSupport.lvclass">)  [unwired: 8 in]
        n93 = Bundle By Name(cluster=w265, "PostBuildSupport"=w262) -> (w266:T3)
        n94 = call <vilib>:"Add State(s) to Queue__JKI_lib_State_Machine.vi"("State(s) in (\"\")"=w268) -> ("States Out"=w267:string)  [unwired: 14 in]
      }
      frame "Build: Copy 7zSD" {
        # "copy 7ZS2.sfx"
        # "copy 7ZS2.sfx"
        n95 = Unbundle By Name(w273) -> ("PostBuildSupport"=w271:refnum<class "PostBuildSupport.lvclass">)
        n96 = call "Copy 7zSD.SFX.vi"("error in (no error)"=w269, "PostBuildSupport in"=w271) -> ("error out"=w272:errorcluster, "PostBuildSupport out"=w270:refnum<class "PostBuildSupport.lvclass">)  [unwired: 8 in]
        n97 = Bundle By Name(cluster=w273, "PostBuildSupport"=w270) -> (w274:T3)
        n98 = call <vilib>:"Add State(s) to Queue__JKI_lib_State_Machine.vi"("State(s) in (\"\")"=w276) -> ("States Out"=w275:string)  [unwired: 14 in]
      }
      frame "Build: Load LV Project" {
        # "find project and open\nbuild specifications"
        # "Template Separator\n(You can make a copy of, or modify, this frame)"
        n99 = Unbundle By Name(w281) -> ("PostBuildSupport"=w280:refnum<class "PostBuildSupport.lvclass">)
        n100 = call "Open Project.vi"("error in (no error)"=w277, "PostBuildSupport in"=w280) -> ("error out"=w278:errorcluster, "PostBuildSupport out"=w279:refnum<class "PostBuildSupport.lvclass">)  [unwired: 8 in]
        n101 = Bundle By Name(cluster=w281, "PostBuildSupport"=w279) -> (w282:T3)
        n102 = call <vilib>:"Add State(s) to Queue__JKI_lib_State_Machine.vi"("State(s) in (\"\")"=w284) -> ("States Out"=w283:string)  [unwired: 14 in]
      }
      frame "Build: Update Build Version" {
        # "update application\nbuild version"
        # "Template Separator\n(You can make a copy of, or modify, this frame)"
        n103 = Unbundle By Name(w289) -> ("PostBuildSupport"=w288:refnum<class "PostBuildSupport.lvclass">)
        n104 = call "Update Build Version.vi"("error in (no error)"=w286, "PostBuildSupport in"=w288) -> ("error out"=w287:errorcluster, "PostBuildSupport out"=w285:refnum<class "PostBuildSupport.lvclass">)  [unwired: 8 in]
        n105 = Bundle By Name(cluster=w289, "PostBuildSupport"=w285) -> (w290:T3)
        n106 = call <vilib>:"Add State(s) to Queue__JKI_lib_State_Machine.vi"("State(s) in (\"\")"=w292) -> ("States Out"=w291:string)  [unwired: 14 in]
      }
      frame "Build: Build Application" {
        # "build exe"
        # "Template Separator\n(You can make a copy of, or modify, this frame)"
        n107 = Unbundle By Name(w297) -> ("PostBuildSupport"=w293:refnum<class "PostBuildSupport.lvclass">)
        n108 = call "Build Application with API.vi"("error in (no error)"=w294, "PostBuildSupport in"=w293) -> ("error out"=w296:errorcluster, "PostBuildSupport out"=w295:refnum<class "PostBuildSupport.lvclass">)  [unwired: 8 in]
        n109 = Bundle By Name(cluster=w297, "PostBuildSupport"=w295) -> (w298:T3)
        n110 = call <vilib>:"Add State(s) to Queue__JKI_lib_State_Machine.vi"("State(s) in (\"\")"=w300) -> ("States Out"=w299:string)  [unwired: 14 in]
      }
      frame "Build: Build Installer" {
        # "build installer"
        # "Template Separator\n(You can make a copy of, or modify, this frame)"
        n111 = Unbundle By Name(w305) -> ("PostBuildSupport"=w304:refnum<class "PostBuildSupport.lvclass">)
        n112 = call "Build Installer.vi"("error in (no error)"=w302, "PostBuildSupport in"=w304) -> ("error out"=w301:errorcluster, "PostBuildSupport out"=w303:refnum<class "PostBuildSupport.lvclass">)  [unwired: 8 in]
        n113 = Bundle By Name(cluster=w305, "PostBuildSupport"=w303) -> (w306:T3)
        n114 = call <vilib>:"Add State(s) to Queue__JKI_lib_State_Machine.vi"("State(s) in (\"\")"=w308) -> ("States Out"=w307:string)  [unwired: 14 in]
      }
      frame "Build: Write 7z Config" {
        # "7z config.txt"
        # "Template Separator\n(You can make a copy of, or modify, this frame)"
        n115 = Unbundle By Name(w313) -> ("PostBuildSupport"=w312:refnum<class "PostBuildSupport.lvclass">)
        n116 = call "Write 7z config.vi"("error in (no error)"=w310, "PostBuildSupport in"=w312) -> ("error out"=w311:errorcluster, "PostBuildSupport out"=w309:refnum<class "PostBuildSupport.lvclass">)  [unwired: 8 in]
        n117 = Bundle By Name(cluster=w313, "PostBuildSupport"=w309) -> (w314:T3)
        n118 = call <vilib>:"Add State(s) to Queue__JKI_lib_State_Machine.vi"("State(s) in (\"\")"=w316) -> ("States Out"=w315:string)  [unwired: 14 in]
      }
      frame "Build: Write 7z" {
        # "write 7z.bat"
        # "Template Separator\n(You can make a copy of, or modify, this frame)"
        n119 = Unbundle By Name(w321) -> ("PostBuildSupport"=w319:refnum<class "PostBuildSupport.lvclass">)
        n120 = call "Write 7z.bat.vi"("error in (no error)"=w317, "PostBuildSupport in"=w319) -> ("error out"=w320:errorcluster, "PostBuildSupport out"=w318:refnum<class "PostBuildSupport.lvclass">)  [unwired: 8 in]
        n121 = Bundle By Name(cluster=w321, "PostBuildSupport"=w318) -> (w322:T3)
        n122 = call <vilib>:"Add State(s) to Queue__JKI_lib_State_Machine.vi"("State(s) in (\"\")"=w324) -> ("States Out"=w323:string)  [unwired: 14 in]
      }
      frame "Build: Execute 7z" {
        # "execute .bat"
        # "Template Separator\n(You can make a copy of, or modify, this frame)"
        n123 = Unbundle By Name(w329) -> ("PostBuildSupport"=w328:refnum<class "PostBuildSupport.lvclass">)
        n124 = call "Execute 7z bat.vi"("error in (no error)"=w326, "PostBuildSupport in"=w328) -> ("error out"=w327:errorcluster, "PostBuildSupport out"=w325:refnum<class "PostBuildSupport.lvclass">)  [unwired: 8 in]
        n125 = Bundle By Name(cluster=w329, "PostBuildSupport"=w325) -> (w330:T3)
        n126 = call <vilib>:"Add State(s) to Queue__JKI_lib_State_Machine.vi"("State(s) in (\"\")"=w332) -> ("States Out"=w331:string)  [unwired: 14 in]
      }
    }
  }
  "error out" <- w1
